vi "4. 生成：管道内的 光纤分布 数组.vi"(0 "光纤起点":dbl[](array[numeric])) -> (7 "光纤分布":dbl[][](array[numeric]))   [LabVIEW 2018]
uses:
  67cf5c7d-4b33-4dba-b3e5-b9b6b0395875.vi
  ecebee2e-6ce9-4250-8460-20675c2ffb92.vi
  7d41fd3f-bdf0-4fdb-9055-0b81537847c6.vi
  106388a1-76b2-417b-a9d3-1da43cf7a4e9.vi
  42368193-51a0-45c9-a1e2-7c4b12e1721c.vi
  97a8c2cc-7000-43b7-b166-aab71b4ab13a.vi
  f3128a6f-0bbe-4d19-9b62-e77b6ac90e92.vi
  51b0af45-2ce2-4495-9bfd-0a072661e875.vi
  2e1e858f-a0c9-4d26-9584-8770dc7802fa.vi
  9fa2a156-3f2c-472d-b596-9e68b2bff53f.vi
  4424169a-8e1b-4a03-8265-c96e8ab7444b.vi
  cccbceeb-be56-4cb2-b551-805860b94004.vi
  249e5e63-1c1d-47ec-b199-5f19e4438805.vi
  8015abea-76ab-4c38-93f2-4665ae15019e.vi
  7fb39498-c4ba-4aaf-924e-c9966a1e7e9f.vi
  61a5e225-0b8e-438e-b9a9-5d8b150e0e72.vi
  bcbd6dee-7ae5-46ce-a43d-cf87bda8af75.vi
  0a7a0f65-44ee-44d7-a518-52834c7b70db.vi
  c6e16e0a-9f8d-4311-8f94-15ca95066509.vi
  d2fa4bd1-7364-4e19-bcf1-b22e029261a3.vi
  70a51656-fa34-4212-9f21-11cce5834fb2.vi
  c7c54753-fae6-4bed-84cd-68a5bf9ebef1.vi
  6c3abbeb-1155-43d3-b8e5-20b1646dd922.vi
  38cdcb18-f350-42bb-b15c-62178094d3ee.vi
  82b05684-183c-45be-92d2-f099c349b210.vi
  d1d982d3-423b-4c90-b46b-a6753e5f51c7.vi
  53de5f26-a082-472a-923b-abb7920cbd30.vi
  65522db7-aec0-4dbf-8e79-11c6ce7497d3.vi
  828ace54-1579-4710-94c0-2ffb10f453fb.vi
  3a0a4d87-f9cd-49dd-97c5-92d7860d5142.vi
  68d10531-d9b5-4ce6-ac84-aa681663b177.vi
  25d71293-f93c-474c-8577-2579c555340d.vi
  7eea9c6b-0116-442f-904a-3ca4d77bbae7.vi
  899b2014-1212-4ad1-bdf8-2b620fb32715.vi
  d1954f89-634f-40e8-aaef-6c2b821688da.vi
  819a09ce-3d6d-41b9-bb16-d817917edff7.vi
  0ca36df2-680a-49b0-865d-75b09fc2474e.vi
  e3a68484-6bb2-4aed-b23d-06d5e58c82cb.vi
  b7c86ea7-f4dc-4461-9301-47afb4ef5e81.vi
  0afe329b-62be-4c54-b886-ac8209ab9e65.vi
  6aad7102-b981-44fb-8d61-3354c6b6d53b.vi
  28382d43-7fb8-46b6-ad6f-2a4f83859944.vi
  9f6c985e-1d26-487f-a82a-97628126152c.vi
  45f3542c-db7e-4199-a54f-511531027e83.vi
  9cf391e0-697d-4ccc-8152-2bfaaa5ea01a.vi
panel:
  in  "初始2维数组，只含 起点":dbl[][](array[numeric])
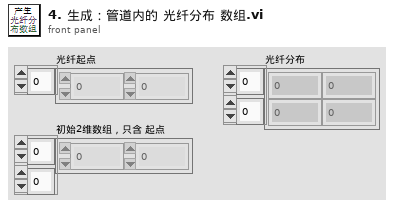
[diagram p1: front panel]
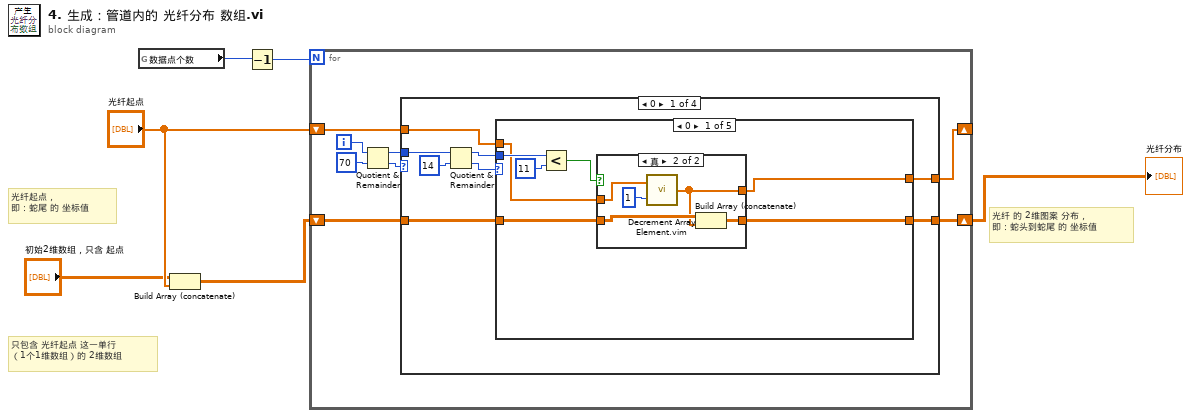
[diagram p0: block diagram]
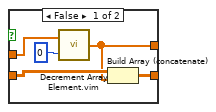
[diagram p2: hidden frame]
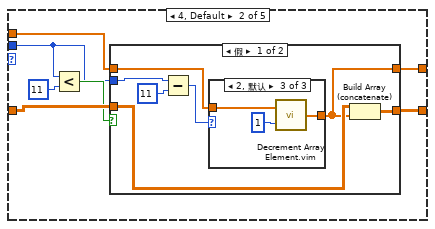
[diagram p3: hidden frame]
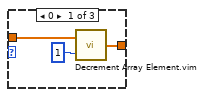
[diagram p4: hidden frame]
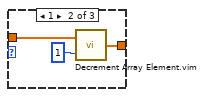
[diagram p5: hidden frame]
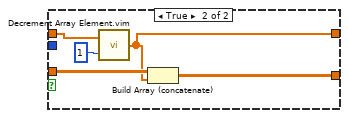
[diagram p6: hidden frame]
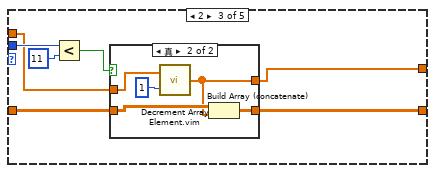
[diagram p7: hidden frame]
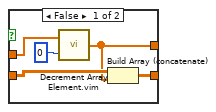
[diagram p8: hidden frame]
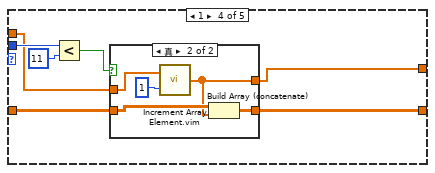
[diagram p9: hidden frame]
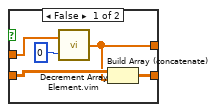
[diagram p10: hidden frame]
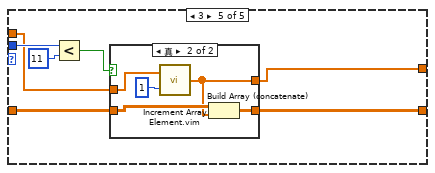
[diagram p11: hidden frame]
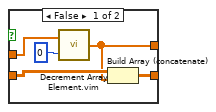
[diagram p12: hidden frame]
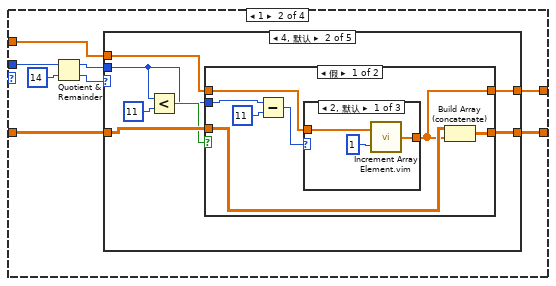
[diagram p13: hidden frame]
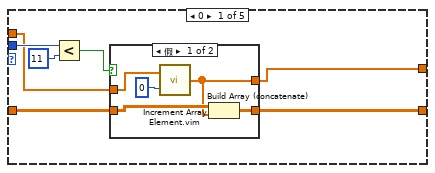
[diagram p14: hidden frame]
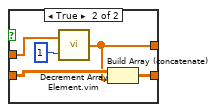
[diagram p15: hidden frame]
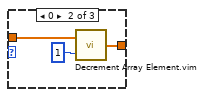
[diagram p16: hidden frame]
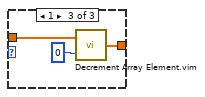
[diagram p17: hidden frame]
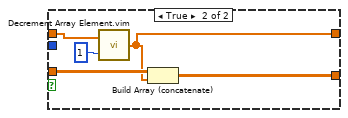
[diagram p18: hidden frame]
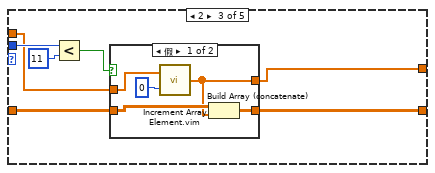
[diagram p19: hidden frame]
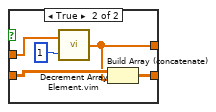
[diagram p20: hidden frame]
diagram:
  # "只包含 光纤起点 这一单行\n（1个1维数组）的 2维数组"
  # "光纤 的 2维图案 分布，\n即：蛇头到蛇尾 的 坐标值"
  # "光纤起点，\n即：蛇尾 的 坐标值"
  n1 = global read "全局变量：数据点个数.vi" "数据点个数"() -> (w2:i32)
  n2 = Build Array (concatenate)("初始2维数组，只含 起点", "光纤起点") -> (w5:dbl[][])
  n3 = Decrement(x=w2) -> (x-1=w1:i32)
  n4 = for {
    N: w1 -> [_]
    shift-right: [w9] -> _
    shift-left: "光纤起点" -> [w10]
    shift-right: [w7] -> w3
    shift-left: w5 -> [w8]
    i -> [w14]
    n5 = Quotient & Remainder(x=w14, y=70) -> (x-y*floor(x/y)=w11:i32, floor(x/y)=w13:i32)
    n6 = case shown="0" w13 {
      tunnel: w11 -> [w22 w126 w230 w334]
      tunnel: w10 -> [w18 w122 w226 w330]
      tunnel: [w17 w121 w225 w329] -> w9
      tunnel: w8 -> [w16 w120 w224 w328]
      tunnel: [w15 w119 w223 w327] -> w7
      frame 0 {
        n7 = Quotient & Remainder(x=w22, y=14) -> (x-y*floor(x/y)=w19:i32, floor(x/y)=w20:i32)
        n8 = case shown="0" w20 {
          tunnel: w19 -> [w29 w40 w74 w91 w108]
          tunnel: w18 -> [w27 w45 w72 w89 w106]
          tunnel: [w26 w44 w71 w88 w105] -> w17
          tunnel: w16 -> [w25 w43 w70 w87 w104]
          tunnel: [w24 w42 w69 w86 w103] -> w15
          frame 0 {
            n9 = Less?(x=w29, y=11) -> (x < y?=w23:bool)
            n10 = case shown="真" w23 {
              tunnel: w27 -> [w31 w36]
              tunnel: [w30 w35] -> w26
              tunnel: w25 -> [w34 w39]
              tunnel: [w33 w38] -> w24
              frame False {
                n11 = call "Decrement Array Element.vim"("index"=0, "array in"=w31) -> ("array out"=w30:dbl[])
                n12 = Build Array (concatenate)(w34, w30) -> (w33:dbl[][])
              }
              frame True {
                n13 = call "Decrement Array Element.vim"("index"=1, "array in"=w36) -> ("array out"=w35:dbl[])
                n14 = Build Array (concatenate)(w39, w35) -> (w38:dbl[][])
              }
            }
          }
          frame 4, Default {
            n15 = Less?(x=w40, y=11) -> (x < y?=w41:bool)
            n16 = case shown="假" w41 {
              tunnel: w45 -> [w48 w64]
              tunnel: [w47 w63] -> w44
              tunnel: w43 -> [w53 w67]
              tunnel: [w52 w66] -> w42
              tunnel: w40 -> [w51 _]
              frame False {
                n17 = Subtract(x=w51, y=11) -> (x-y=w49:i32)
                n18 = case shown="2, 默认" w49 {
                  tunnel: w48 -> [w55 w57 w60]
                  tunnel: [w54 w59 w62] -> w47
                  frame 0 {
                    n19 = call "Decrement Array Element.vim"("index"=1, "array in"=w55) -> ("array out"=w54:dbl[])
                  }
                  frame 1 {
                    n20 = call "Decrement Array Element.vim"("index"=1, "array in"=w57) -> ("array out"=w59:dbl[])
                  }
                  frame 2, Default {
                    n21 = call "Decrement Array Element.vim"("index"=1, "array in"=w60) -> ("array out"=w62:dbl[])
                  }
                }
                n22 = Build Array (concatenate)(w53, w47) -> (w52:dbl[][])
              }
              frame True {
                n23 = call "Decrement Array Element.vim"("index"=1, "array in"=w64) -> ("array out"=w63:dbl[])
                n24 = Build Array (concatenate)(w67, w63) -> (w66:dbl[][])
              }
            }
          }
          frame 2 {
            n25 = Less?(x=w74, y=11) -> (x < y?=w68:bool)
            n26 = case shown="真" w68 {
              tunnel: w72 -> [w76 w81]
              tunnel: [w75 w80] -> w71
              tunnel: w70 -> [w79 w84]
              tunnel: [w78 w83] -> w69
              frame False {
                n27 = call "Decrement Array Element.vim"("index"=0, "array in"=w76) -> ("array out"=w75:dbl[])
                n28 = Build Array (concatenate)(w79, w75) -> (w78:dbl[][])
              }
              frame True {
                n29 = call "Decrement Array Element.vim"("index"=1, "array in"=w81) -> ("array out"=w80:dbl[])
                n30 = Build Array (concatenate)(w84, w80) -> (w83:dbl[][])
              }
            }
          }
          frame 1 {
            n31 = Less?(x=w91, y=11) -> (x < y?=w85:bool)
            n32 = case shown="真" w85 {
              tunnel: w89 -> [w93 w99]
              tunnel: [w92 w97] -> w88
              tunnel: w87 -> [w96 w101]
              tunnel: [w95 w100] -> w86
              frame False {
                n33 = call "Decrement Array Element.vim"("index"=0, "array in"=w93) -> ("array out"=w92:dbl[])
                n34 = Build Array (concatenate)(w96, w92) -> (w95:dbl[][])
              }
              frame True {
                n35 = call "Increment Array Element.vim"("index"=1, "array in"=w99) -> ("array out"=w97:dbl[])
                n36 = Build Array (concatenate)(w101, w97) -> (w100:dbl[][])
              }
            }
          }
          frame 3 {
            n37 = Less?(x=w108, y=11) -> (x < y?=w102:bool)
            n38 = case shown="真" w102 {
              tunnel: w106 -> [w110 w116]
              tunnel: [w109 w114] -> w105
              tunnel: w104 -> [w113 w118]
              tunnel: [w112 w117] -> w103
              frame False {
                n39 = call "Decrement Array Element.vim"("index"=0, "array in"=w110) -> ("array out"=w109:dbl[])
                n40 = Build Array (concatenate)(w113, w109) -> (w112:dbl[][])
              }
              frame True {
                n41 = call "Increment Array Element.vim"("index"=1, "array in"=w116) -> ("array out"=w114:dbl[])
                n42 = Build Array (concatenate)(w118, w114) -> (w117:dbl[][])
              }
            }
          }
        }
      }
      frame 1 {
        n43 = Quotient & Remainder(x=w126, y=14) -> (x-y*floor(x/y)=w123:i32, floor(x/y)=w124:i32)
        n44 = case shown="4, 默认" w124 {
          tunnel: w123 -> [w133 w144 w178 w195 w212]
          tunnel: w122 -> [w131 w149 w176 w193 w210]
          tunnel: [w130 w148 w175 w192 w209] -> w121
          tunnel: w120 -> [w129 w147 w174 w191 w208]
          tunnel: [w128 w146 w173 w190 w207] -> w119
          frame 0 {
            n45 = Less?(x=w133, y=11) -> (x < y?=w127:bool)
            n46 = case shown="假" w127 {
              tunnel: w131 -> [w135 w140]
              tunnel: [w134 w139] -> w130
              tunnel: w129 -> [w138 w143]
              tunnel: [w137 w142] -> w128
              frame False {
                n47 = call "Increment Array Element.vim"("index"=0, "array in"=w135) -> ("array out"=w134:dbl[])
                n48 = Build Array (concatenate)(w138, w134) -> (w137:dbl[][])
              }
              frame True {
                n49 = call "Decrement Array Element.vim"("index"=1, "array in"=w140) -> ("array out"=w139:dbl[])
                n50 = Build Array (concatenate)(w143, w139) -> (w142:dbl[][])
              }
            }
          }
          frame 4, Default {
            n51 = Less?(x=w144, y=11) -> (x < y?=w145:bool)
            n52 = case shown="假" w145 {
              tunnel: w149 -> [w152 w168]
              tunnel: [w151 w167] -> w148
              tunnel: w147 -> [w157 w171]
              tunnel: [w156 w170] -> w146
              tunnel: w144 -> [w154 _]
              frame False {
                n53 = Subtract(x=w154, y=11) -> (x-y=w153:i32)
                n54 = case shown="2, 默认" w153 {
                  tunnel: w152 -> [w160 w161 w164]
                  tunnel: [w158 w162 w165] -> w151
                  frame 2, Default {
                    n55 = call "Increment Array Element.vim"("index"=1, "array in"=w160) -> ("array out"=w158:dbl[])
                  }
                  frame 0 {
                    n56 = call "Decrement Array Element.vim"("index"=1, "array in"=w161) -> ("array out"=w162:dbl[])
                  }
                  frame 1 {
                    n57 = call "Decrement Array Element.vim"("index"=0, "array in"=w164) -> ("array out"=w165:dbl[])
                  }
                }
                n58 = Build Array (concatenate)(w157, w151) -> (w156:dbl[][])
              }
              frame True {
                n59 = call "Decrement Array Element.vim"("index"=1, "array in"=w168) -> ("array out"=w167:dbl[])
                n60 = Build Array (concatenate)(w171, w167) -> (w170:dbl[][])
              }
            }
          }
          frame 2 {
            n61 = Less?(x=w178, y=11) -> (x < y?=w172:bool)
            n62 = case shown="假" w172 {
              tunnel: w176 -> [w179 w185]
              tunnel: [w180 w184] -> w175
              tunnel: w174 -> [w183 w188]
              tunnel: [w182 w187] -> w173
              frame False {
                n63 = call "Increment Array Element.vim"("index"=0, "array in"=w179) -> ("array out"=w180:dbl[])
                n64 = Build Array (concatenate)(w183, w180) -> (w182:dbl[][])
              }
              frame True {
                n65 = call "Decrement Array Element.vim"("index"=1, "array in"=w185) -> ("array out"=w184:dbl[])
                n66 = Build Array (concatenate)(w188, w184) -> (w187:dbl[][])
              }
            }
          }
          frame 1 {
            n67 = Less?(x=w195, y=11) -> (x < y?=w189:bool)
            n68 = case shown="假" w189 {
              tunnel: w193 -> [w196 w203]
              tunnel: [w197 w201] -> w192
              tunnel: w191 -> [w200 w205]
              tunnel: [w199 w204] -> w190
              frame False {
                n69 = call "Increment Array Element.vim"("index"=0, "array in"=w196) -> ("array out"=w197:dbl[])
                n70 = Build Array (concatenate)(w200, w197) -> (w199:dbl[][])
              }
              frame True {
                n71 = call "Increment Array Element.vim"("index"=1, "array in"=w203) -> ("array out"=w201:dbl[])
                n72 = Build Array (concatenate)(w205, w201) -> (w204:dbl[][])
              }
            }
          }
          frame 3 {
            n73 = Less?(x=w212, y=11) -> (x < y?=w206:bool)
            n74 = case shown="假" w206 {
              tunnel: w210 -> [w213 w220]
              tunnel: [w215 w218] -> w209
              tunnel: w208 -> [w217 w222]
              tunnel: [w216 w221] -> w207
              frame False {
                n75 = call "Increment Array Element.vim"("index"=0, "array in"=w213) -> ("array out"=w215:dbl[])
                n76 = Build Array (concatenate)(w217, w215) -> (w216:dbl[][])
              }
              frame True {
                n77 = call "Increment Array Element.vim"("index"=1, "array in"=w220) -> ("array out"=w218:dbl[])
                n78 = Build Array (concatenate)(w222, w218) -> (w221:dbl[][])
              }
            }
          }
        }
      }
      frame 2 {
        n79 = Quotient & Remainder(x=w230, y=14) -> (x-y*floor(x/y)=w227:i32, floor(x/y)=w228:i32)
        n80 = case shown="4, 默认" w228 {
          tunnel: w227 -> [w237 w248 w282 w299 w316]
          tunnel: w226 -> [w235 w253 w280 w297 w314]
          tunnel: [w234 w252 w279 w296 w313] -> w225
          tunnel: w224 -> [w233 w251 w278 w295 w312]
          tunnel: [w232 w250 w277 w294 w311] -> w223
          frame 0 {
            n81 = Less?(x=w237, y=11) -> (x < y?=w231:bool)
            n82 = case shown="真" w231 {
              tunnel: w235 -> [w239 w244]
              tunnel: [w238 w243] -> w234
              tunnel: w233 -> [w242 w247]
              tunnel: [w241 w246] -> w232
              frame False {
                n83 = call "Increment Array Element.vim"("index"=1, "array in"=w239) -> ("array out"=w238:dbl[])
                n84 = Build Array (concatenate)(w242, w238) -> (w241:dbl[][])
              }
              frame True {
                n85 = call "Decrement Array Element.vim"("index"=0, "array in"=w244) -> ("array out"=w243:dbl[])
                n86 = Build Array (concatenate)(w247, w243) -> (w246:dbl[][])
              }
            }
          }
          frame 4, Default {
            n87 = Less?(x=w248, y=11) -> (x < y?=w249:bool)
            n88 = case shown="假" w249 {
              tunnel: w253 -> [w257 w272]
              tunnel: [w256 w271] -> w252
              tunnel: w251 -> [w261 w275]
              tunnel: [w260 w274] -> w250
              tunnel: w248 -> [w259 _]
              frame False {
                n89 = Subtract(x=w259, y=11) -> (x-y=w255:i32)
                n90 = case shown="2, 默认" w255 {
                  tunnel: w257 -> [w264 w265 w268]
                  tunnel: [w262 w267 w270] -> w256
                  frame 0 {
                    n91 = call "Decrement Array Element.vim"("index"=0, "array in"=w264) -> ("array out"=w262:dbl[])
                  }
                  frame 1 {
                    n92 = call "Increment Array Element.vim"("index"=1, "array in"=w265) -> ("array out"=w267:dbl[])
                  }
                  frame 2, Default {
                    n93 = call "Increment Array Element.vim"("index"=0, "array in"=w268) -> ("array out"=w270:dbl[])
                  }
                }
                n94 = Build Array (concatenate)(w261, w256) -> (w260:dbl[][])
              }
              frame True {
                n95 = call "Decrement Array Element.vim"("index"=0, "array in"=w272) -> ("array out"=w271:dbl[])
                n96 = Build Array (concatenate)(w275, w271) -> (w274:dbl[][])
              }
            }
          }
          frame 2 {
            n97 = Less?(x=w282, y=11) -> (x < y?=w276:bool)
            n98 = case shown="真" w276 {
              tunnel: w280 -> [w283 w289]
              tunnel: [w284 w288] -> w279
              tunnel: w278 -> [w287 w292]
              tunnel: [w286 w291] -> w277
              frame False {
                n99 = call "Increment Array Element.vim"("index"=1, "array in"=w283) -> ("array out"=w284:dbl[])
                n100 = Build Array (concatenate)(w287, w284) -> (w286:dbl[][])
              }
              frame True {
                n101 = call "Decrement Array Element.vim"("index"=0, "array in"=w289) -> ("array out"=w288:dbl[])
                n102 = Build Array (concatenate)(w292, w288) -> (w291:dbl[][])
              }
            }
          }
          frame 1 {
            n103 = Less?(x=w299, y=11) -> (x < y?=w293:bool)
            n104 = case shown="真" w293 {
              tunnel: w297 -> [w300 w307]
              tunnel: [w301 w305] -> w296
              tunnel: w295 -> [w304 w309]
              tunnel: [w303 w308] -> w294
              frame False {
                n105 = call "Increment Array Element.vim"("index"=1, "array in"=w300) -> ("array out"=w301:dbl[])
                n106 = Build Array (concatenate)(w304, w301) -> (w303:dbl[][])
              }
              frame True {
                n107 = call "Increment Array Element.vim"("index"=0, "array in"=w307) -> ("array out"=w305:dbl[])
                n108 = Build Array (concatenate)(w309, w305) -> (w308:dbl[][])
              }
            }
          }
          frame 3 {
            n109 = Less?(x=w316, y=11) -> (x < y?=w310:bool)
            n110 = case shown="真" w310 {
              tunnel: w314 -> [w317 w324]
              tunnel: [w319 w322] -> w313
              tunnel: w312 -> [w321 w326]
              tunnel: [w320 w325] -> w311
              frame False {
                n111 = call "Increment Array Element.vim"("index"=1, "array in"=w317) -> ("array out"=w319:dbl[])
                n112 = Build Array (concatenate)(w321, w319) -> (w320:dbl[][])
              }
              frame True {
                n113 = call "Increment Array Element.vim"("index"=0, "array in"=w324) -> ("array out"=w322:dbl[])
                n114 = Build Array (concatenate)(w326, w322) -> (w325:dbl[][])
              }
            }
          }
        }
      }
      frame 3, Default {
        n115 = Quotient & Remainder(x=w334, y=14) -> (x-y*floor(x/y)=w331:i32, floor(x/y)=w332:i32)
        n116 = case shown="4, 默认" w332 {
          tunnel: w331 -> [w341 w358 w373 w390 w407]
          tunnel: w330 -> [w339 w356 w371 w388 w405]
          tunnel: [w338 w355 w370 w387 w404] -> w329
          tunnel: w328 -> [w337 w354 w369 w386 w403]
          tunnel: [w336 w353 w368 w385 w402] -> w327
          frame 3 {
            n117 = Less?(x=w341, y=11) -> (x < y?=w335:bool)
            n118 = case shown="真" w335 {
              tunnel: w339 -> [w343 w348]
              tunnel: [w342 w347] -> w338
              tunnel: w337 -> [w346 w351]
              tunnel: [w345 w350] -> w336
              frame False {
                n119 = call "Increment Array Element.vim"("index"=1, "array in"=w343) -> ("array out"=w342:dbl[])
                n120 = Build Array (concatenate)(w346, w342) -> (w345:dbl[][])
              }
              frame True {
                n121 = call "Decrement Array Element.vim"("index"=0, "array in"=w348) -> ("array out"=w347:dbl[])
                n122 = Build Array (concatenate)(w351, w347) -> (w350:dbl[][])
              }
            }
          }
          frame 4, Default {
            n123 = Less?(x=w358, y=11) -> (x < y?=w352:bool)
            n124 = case shown="真" w352 {
              tunnel: w356 -> [w359 w363]
              tunnel: [w359 w364] -> w355
              tunnel: w354 -> [w361 w366]
              tunnel: [w360 w365] -> w353
              frame False {
                n125 = Build Array (concatenate)(w361, w359) -> (w360:dbl[][])
              }
              frame True {
                n126 = call "Increment Array Element.vim"("index"=0, "array in"=w363) -> ("array out"=w364:dbl[])
                n127 = Build Array (concatenate)(w366, w364) -> (w365:dbl[][])
              }
            }
          }
          frame 1 {
            n128 = Less?(x=w373, y=11) -> (x < y?=w367:bool)
            n129 = case shown="真" w367 {
              tunnel: w371 -> [w374 w380]
              tunnel: [w375 w379] -> w370
              tunnel: w369 -> [w378 w383]
              tunnel: [w377 w382] -> w368
              frame False {
                n130 = call "Increment Array Element.vim"("index"=1, "array in"=w374) -> ("array out"=w375:dbl[])
                n131 = Build Array (concatenate)(w378, w375) -> (w377:dbl[][])
              }
              frame True {
                n132 = call "Decrement Array Element.vim"("index"=0, "array in"=w380) -> ("array out"=w379:dbl[])
                n133 = Build Array (concatenate)(w383, w379) -> (w382:dbl[][])
              }
            }
          }
          frame 0 {
            n134 = Less?(x=w390, y=11) -> (x < y?=w384:bool)
            n135 = case shown="真" w384 {
              tunnel: w388 -> [w391 w398]
              tunnel: [w392 w396] -> w387
              tunnel: w386 -> [w395 w400]
              tunnel: [w394 w399] -> w385
              frame False {
                n136 = call "Increment Array Element.vim"("index"=1, "array in"=w391) -> ("array out"=w392:dbl[])
                n137 = Build Array (concatenate)(w395, w392) -> (w394:dbl[][])
              }
              frame True {
                n138 = call "Increment Array Element.vim"("index"=0, "array in"=w398) -> ("array out"=w396:dbl[])
                n139 = Build Array (concatenate)(w400, w396) -> (w399:dbl[][])
              }
            }
          }
          frame 2 {
            n140 = Less?(x=w407, y=11) -> (x < y?=w401:bool)
            n141 = case shown="真" w401 {
              tunnel: w405 -> [w408 w415]
              tunnel: [w410 w413] -> w404
              tunnel: w403 -> [w412 w417]
              tunnel: [w411 w416] -> w402
              frame False {
                n142 = call "Increment Array Element.vim"("index"=1, "array in"=w408) -> ("array out"=w410:dbl[])
                n143 = Build Array (concatenate)(w412, w410) -> (w411:dbl[][])
              }
              frame True {
                n144 = call "Increment Array Element.vim"("index"=0, "array in"=w415) -> ("array out"=w413:dbl[])
                n145 = Build Array (concatenate)(w417, w413) -> (w416:dbl[][])
              }
            }
          }
        }
      }
    }
  }
  "光纤分布" <- w3
